vi "LEP_RV_OCDIOptionsDlg.vi"   [LabVIEW 2011]
doc: "Map menu items to commands."
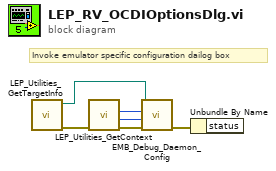
[diagram p0: block diagram]
diagram:
  # "Invoke emulator specific configuration dailog box"
  n1 = call <vilib>:"LEP_Utilities_GetTargetInfo.vi"() -> ("error out"=w4:errorcluster, "path"=w5:path)  [unwired: 8 in, 2 out]
  n2 = call <vilib>:"LEP_Utilities_GetContext.vi"("error in"=w4) -> ("error out"=w3:errorcluster, "build ID"=w1:u32, "target ID"=w2:u32)  [unwired: 7 in, 1 out]
  n3 = call <vilib>:"EMB_Debug_Daemon_Config.vi"("error in (no error)"=w3, "build ID"=w1, "target ID"=w2, "target path"=w5) -> ("error out"=w6:errorcluster)  [unwired: 7 in]
  n4 = Unbundle By Name(w6) -> ()  [unwired: 1 out]
